vi "Proj1_frontpanel.vi"() -> ()   [LabVIEW 2022 SP3]
panel:
  out "Waveform Chart":dbl(graph)
  in  "stop":bool
  out "Numeric 3":dbl
  in  "Numeric 2":dbl
  in  "Numeric":dbl
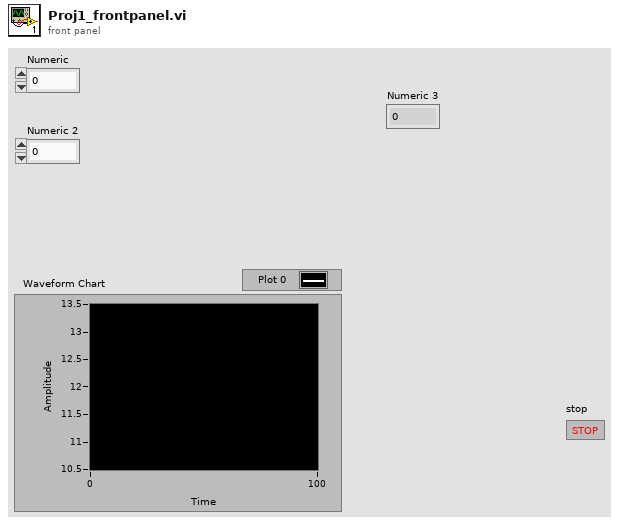
[diagram p1: front panel]
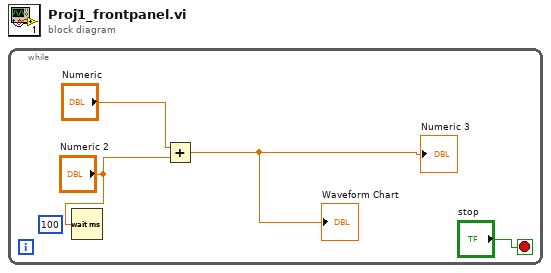
[diagram p0: block diagram]
diagram:
  n1 = while {
    stop <- "stop" stop-if-true
    (unwired) u32 100 ("milliseconds to wait")
    n2 = Wait (ms)(milliseconds to wait="Numeric 2") -> ()  [unwired: 1 out]
    n3 = Add(x="Numeric", y="Numeric 2") -> (x+y=→"Numeric 3" →"Waveform Chart":dbl)
  }
